vi "SerialGetXSpeed.vi"(2 "error in (no error)":errorcluster) -> (0 "error out":errorcluster, 1 "Speed mm/sec":dbl)   [LabVIEW 2010]
panel:
  in  "Command prefix in":string="1H"
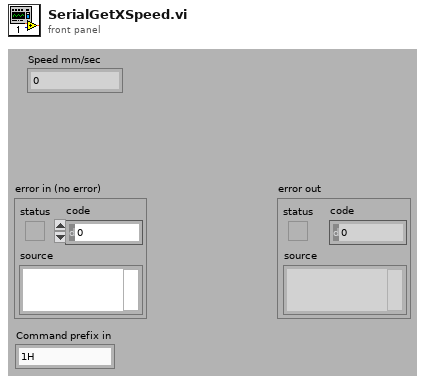
[diagram p1: front panel]
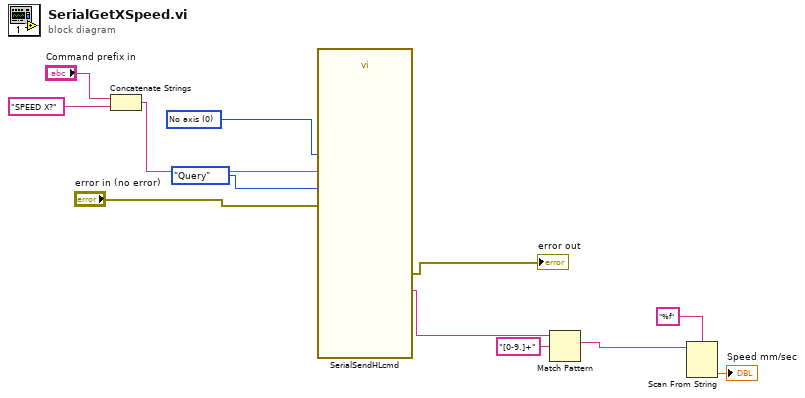
[diagram p0: block diagram]
diagram:
  w8 = u16 0 items=["No axis", "X", "Y", "Z", "XY", "XYZ"] ("Axis configuration")
  n1 = Concatenate Strings("Command prefix in", "SPEED X?" ("Command")) -> (w2:string)
  n2 = call "SerialSendHLcmd.vi"("Command"=w2, "Axis configuration"=w8, "error in (no error)"="error in (no error)", "Command type"=enum16{"Query", "Where", "Imperative", "DU Y"}."Query") -> ("Raw receive buffer"=w1:string, "error out"=→"error out":errorcluster)  [unwired: 7 in, 3 out]
  n3 = Match Pattern(string=w1, regular expression="[0-9.]+") -> (match substring=w11:string)  [unwired: 1 in, 3 out]
  n4 = Scan From String "Scan From String"(format string="%f", input string=w11) -> (output 1=→"Speed mm/sec":dbl)  [unwired: 3 in, 3 out]
